vi "setUp.vi"(8 "error in (no error)":errorcluster, 11 "reference in":refnum<class "Routing and Faulting Validation Unit Tests.lvclass">) -> (0 "error out":errorcluster, 3 "reference out":refnum<class "Routing and Faulting Validation Unit Tests.lvclass">)   [LabVIEW 2019, in "Routing and Faulting Validation Unit Tests.lvclass"]
doc: "setUp runs prior to the test method during test execution. Use this method to initialize any object data required by your tests."
uses:
  Routing and Faulting Validation Unit Tests.lvclass
  C:/Program Files (x86)/National Instruments/LabVIEW 2019/vi.lib/addons/_JKI Toolkits/VI Tester/TestCase.llb/TestCase.lvclass
  NationalInstruments.VeriStand.SystemDefinitionAPI
  Routing and Faulting Validation Unit Tests.lvclass/Routing and Faulting Validation Unit Tests.ctl
  <userlib>/_OpenG.lib/file/file.llb/Append Path to Root if Relative - Scalar__ogtk.vi
  <vilib>/addons/_JKI Toolkits/VI Tester/TestCase.llb/TestCase.lvclass
  niveristand-custom-device-testing-tools/VeriStandTestUtilities/VeriStandTestUtilities.lvlib
  Routing and Faulting Scripting.lvlib
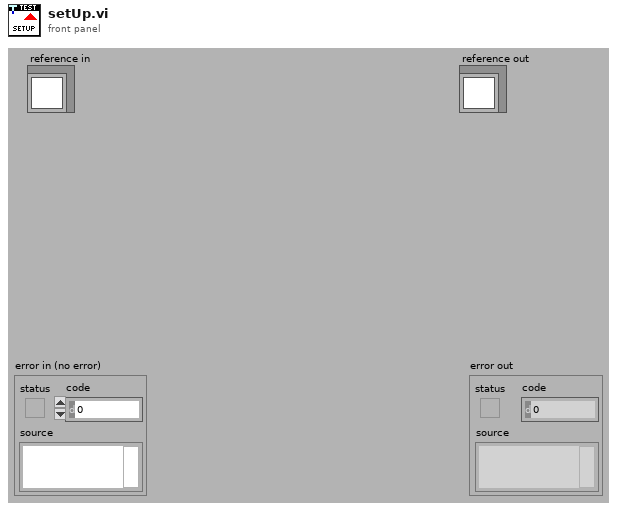
[diagram p1: front panel]
types:
  T1 = typedef "Custom Device API.lvlib/Custom Device Item Ref.ctl" = u64
  T2 = typedef "Routing and Faulting Scripting.lvlib/Module Information.ctl" = cluster{"Module Path":string, "Product Name":string, "Possible Connections":T3[], "Configuration Revision":u32, "Validated":bool, "Missing":bool}
  T3 = typedef "Routing and Faulting Hardware API.lvlib/Possible Connections for Endpoint.ctl" = cluster{"Source":string, "Destinations":string[]}
  T4 = typedef "Routing and Faulting Scripting.lvlib/Validation Information.ctl" = cluster{"Missing Modules":variant, "Module Connection Map":variant, "Unused Modules":variant}
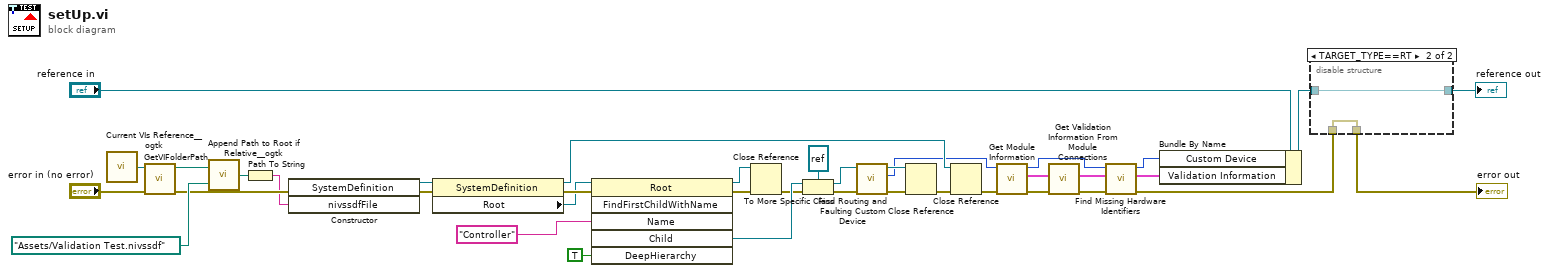
[diagram p0: block diagram]
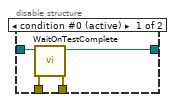
[diagram p2: hidden frame]
diagram:
  n1 = call <userlib>:"Current VIs Reference__ogtk.vi"() -> ("Current VI's reference"=w36:refnum<vi>)  [unwired: 5 in]
  n2 = call "GetVIFolderPath.vi"("error in (no error)"="error in (no error)", "VI Reference in"=w36) -> ("error out"=w32:errorcluster, "VI Folder Path out"=w35:path)  [unwired: 8 in]
  n3 = call-poly <userlib>:"Append Path to Root if Relative__ogtk.vi"("Absolute or Relative Path"=path "Assets/Validation Test.nivssdf", "Root Path"=w35) -> ("Absolute or Appended Path"=w33:path)
  n4 = Path To String(path=w33) -> (string=w30:string)
  n5 = constructor class="SystemDefinition"(error in=w32, "nivssdfFile"=w30) -> (reference out=w29:refnum<k24>, error out=w31:errorcluster)  [unwired: 2 in, 2 out]
  n6 = property class="SystemDefinition"(reference=w29, error in=w31) -> (reference out=w9:refnum<k24>, error out=w28:errorcluster, "Root"=w27:refnum<k24>)
  n7 = invoke class="Root" method="FindFirstChildWithName"(reference=w27, error in=w28, "Name"="Controller", "DeepHierarchy"=TRUE) -> (reference out=w20:refnum<k24>, error out=w22:errorcluster, "Child"=w24:refnum<k24>)  [unwired: 2 in, 3 out]
  n8 = Close Reference(reference=w20, error in (no error)=w22) -> (error out=w21:errorcluster)
  n9 = To More Specific Class(target class=refnum<k24> refnum, reference=w24, error in=w21) -> (specific class reference=w18:refnum<k24>, error out=w19:errorcluster)
  n10 = call "Find Routing and Faulting Custom Device.vi"("error in"=w19, "target in"=w18) -> ("error out"=w13:errorcluster, "routing and faulting custom device"=w8:T1, "target out"=w12:refnum<k24>)  [unwired: 7 in]
  n11 = Close Reference(reference=w12, error in (no error)=w13) -> (error out=w11:errorcluster)
  n12 = Close Reference(reference=w9, error in (no error)=w11) -> (error out=w10:errorcluster)
  n13 = call "Get Module Information.vi"("error in"=w10, "routing and faulting in"=w8) -> ("error out"=w15:errorcluster, "module information"=w14:T2[], "routing and faulting out"=w1:T1)  [unwired: 7 in]
  n14 = call "Get Validation Information From Module Connections.vi"("error in"=w15, "module connection information"=w14) -> ("error out"=w6:errorcluster, "validation information"=w5:T4)  [unwired: 8 in]
  n15 = call "Find Missing Hardware Identifiers.vi"("error in"=w6, "validation information in"=w5, "routing and faulting in"=w1) -> ("error out"=w3:errorcluster, "validation information out"=w4:T4, "routing and faulting out"=w2:T1)  [unwired: 5 in, 1 out]
  n16 = Bundle By Name(cluster="reference in", "Custom Device"=w2, "Validation Information"=w4) -> (w16:refnum<class "Routing and Faulting Validation Unit Tests.lvclass">)
  n17 = disable-structure shown="TARGET_TYPE==RT" {
    disable-tunnel: w3 -> [w42 w43]
    disable-tunnel: [w41 w43] -> w38
    disable-tunnel: [w40 w44] -> w37
    disable-tunnel: w16 -> [w39 w44]
    frame condition #0 (active) {
      n18 = call <vilib>:"WaitOnTestComplete.vi"("error in (no error)"=w42, "TestCase in"=w39) -> ("error out"=w41:errorcluster, "TestCase out"=w40:refnum<class "Routing and Faulting Validation Unit Tests.lvclass">)  [unwired: 8 in]
    }
    frame condition #1 {
    }
  }
  "error out" <- w38
  "reference out" <- w37
